vi "Left Camera Loop (SubVI).vi"   [LabVIEW 2015]
uses:
  <vilib>/myRIO/Instrument Drivers/Onboard IO/SPI/typedefs/SPI User Configuration.ctl
  <vilib>/myRIO/Common/Instrument Driver Framework/myRIO v1.0/SPI/typedefs/SPI Clock Phase.ctl
  <vilib>/myRIO/Common/Instrument Driver Framework/myRIO v1.0/SPI/typedefs/SPI Clock Polarity.ctl
  <vilib>/myRIO/Common/Instrument Driver Framework/myRIO v1.0/SPI/typedefs/SPI Data Direction.ctl
  <vilib>/myRIO/Common/Instrument Driver Framework/myRIO v1.0/SPI/typedefs/SPI Frame Length.ctl
  <vilib>/Utility/error.llb/Error Cluster From Error Code.vi
  <vilib>/myRIO/Common/Instrument Driver Framework/myRIO v1.0/SPI/vis/myRIO v1.0 Configure SPI.vi
  Left Variables.vi
  <vilib>/myRIO/Instrument Drivers/Onboard IO/SPI/SPI.lvlib
types:
  T1 = typedef "SPI.lvlib/SPI User Configuration.ctl" = cluster{"Frequency [Hz]":dbl, "Clock Phase":T2, "Clock Polarity":T3, "Data Direction":T4, "Frame Length":T5}
  T2 = typedef "SPI Clock Phase.ctl" = enum8{"Leading", "Trailing"}
  T3 = typedef "SPI Clock Polarity.ctl" = enum8{"Low", "High"}
  T4 = typedef "SPI Data Direction.ctl" = enum8{"Most significant bit first", "Least significant bit first"}
  T5 = typedef "SPI Frame Length.ctl" = u8
  T6 = typedef "SPI.lvlib/SPI Reference.ctl" = cluster{"myRIO Reference":T7, "SPI Channels Enum":T11, "SPI Configuration":T12}
  T7 = typedef "myRIO Generic Hardware Reference.ctl" = cluster{"myRIO Model":T8, "myRIO Hardware Reference":T9}
  T8 = typedef "Hardware Version Enum.ctl" = enum16{"Unknown", "myRIO-1900", "myRIO-1950", "roboRIO"}
  T9 = typedef "myRIO v1.0 Reference.ctl" = cluster{"Generic FPGA Reference":T10, "Allow multiple opens":bool}
  T10 = typedef "Generic FPGA Reference.ctl" = refnum<k20>
  T11 = typedef "SPI Channels Enum.ctl" = enum16{"Not Connected", "A/SPI", "B/SPI", "SPI/SPI"}
  T12 = typedef "SPI.lvlib/SPI Configuration.ctl" = cluster{"Frequency [Hz]":dbl, "Clock Phase":T2, "Clock Polarity":T3, "Data Direction":T4, "Frame Length":T5}
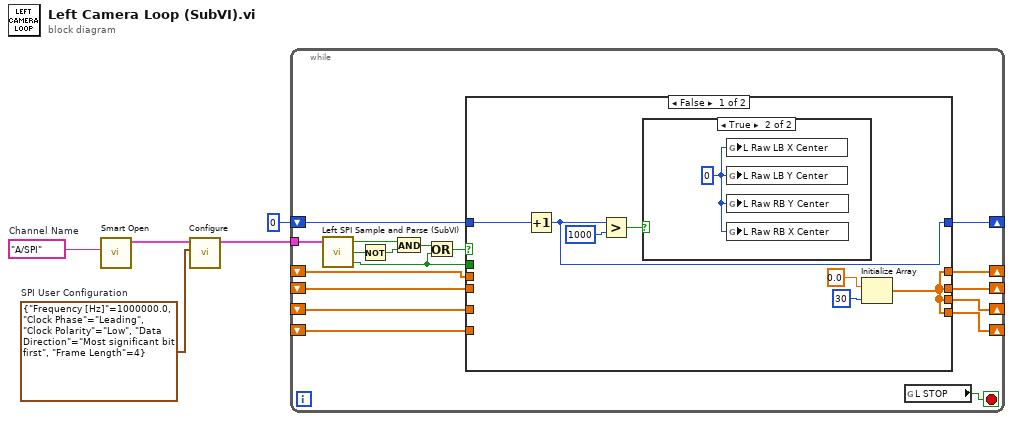
[diagram p0: block diagram]
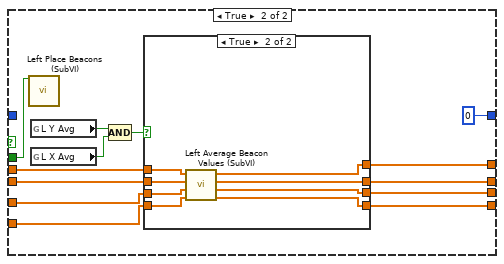
[diagram p3: hidden frame]
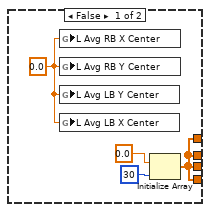
[diagram p4: hidden frame]
diagram:
  w3 = T1 {"Frequency [Hz]"=1000000.0, "Clock Phase"=enum."Leading", "Clock Polarity"=enum."Low", "Data Direction"=enum."Most significant bit first", "Frame Length"=4}  # SPI User Configuration
  w4 = tag "A/SPI"  # Channel Name
  n1 = call <vilib>:"Smart Open.vi"("Channel Name"=w4) -> ("SPI Ref Out"=w2:T6)  [unwired: 9 in, 1 out]
  n2 = call <vilib>:"Configure.vi"("SPI User Configuration"=w3, "SPI Ref In"=w2) -> ("SPI Ref Out"=w1:T6)  [unwired: 8 in, 1 out]
  n3 = while {
    shift-right: [w18] -> _
    shift-left: _ -> [w22]
    shift-right: [w17] -> _
    shift-left: _ -> [w21]
    shift-right: [w16] -> _
    shift-left: _ -> [w20]
    shift-right: [w19] -> _
    shift-left: _ -> [w23]
    shift-right: [w11] -> _
    shift-left: 0 -> [w12]
    tunnel: w1 -> [w9]
    stop <- w10 stop-if-true
    n4 = call "Left SPI Sample and Parse (SubVI).vi"("SPI Ref In"=w9) -> ("Two Beacons Seen?"=w8:bool, "o2 Checksum OK?"=w6:bool, "o1 Checksum OK?"=w7:bool)  [unwired: 2 in]
    n5 = Not(x=w6) -> (.not. x?=w15:bool)
    n6 = And(x=w7, y=w15) -> (x .and. y?=w13:bool)
    n7 = Or(x=w13, y=w8) -> (x .or. y?=w14:bool)
    n8 = case shown="False" w14 {
      tunnel: w23 -> [_ w44]
      tunnel: w22 -> [_ w43]
      tunnel: w21 -> [_ w42]
      tunnel: w20 -> [_ w41]
      tunnel: [w28 w40] -> w19
      tunnel: [w28 w39] -> w18
      tunnel: [w28 w38] -> w17
      tunnel: [w28 w37] -> w16
      tunnel: w8 -> [_ w33]
      tunnel: w12 -> [w26 _]
      tunnel: [w25 0] -> w11
      frame False {
        n9 = Increment(x=w26) -> (x+1=w25:i32)
        n10 = Greater?(x=w25, y=1000) -> (0:w27:bool)
        n11 = case shown="True" w27 {
          frame False {
          }
          frame True {
            w31 = u16 0
            n12 = global write "Left Variables.vi" "L Raw LB X Center"(w31) -> ()
            n13 = global write "Left Variables.vi" "L Raw LB Y Center"(w31) -> ()
            n14 = global write "Left Variables.vi" "L Raw RB Y Center"(w31) -> ()
            n15 = global write "Left Variables.vi" "L Raw RB X Center"(w31) -> ()
          }
        }
        n16 = Initialize Array(0.0 ("element"), 30 ("dimension size")) -> (w28:dbl[])
      }
      frame True {
        n17 = call "Left Place Beacons (SubVI).vi"("Two Beacons Seen"=w33) -> ()  [unwired: 15 in]
        n18 = global read "Left Variables.vi" "L Y Avg"() -> (w36:bool)
        n19 = global read "Left Variables.vi" "L X Avg"() -> (w35:bool)
        n20 = Compound Arithmetic op=AND(w36, w35) -> (w34:bool)
        n21 = case shown="True" w34 {
          tunnel: w44 -> [_ w56]
          tunnel: w43 -> [_ w54]
          tunnel: w42 -> [_ w52]
          tunnel: w41 -> [_ w50]
          tunnel: [w46 w55] -> w40
          tunnel: [w46 w53] -> w39
          tunnel: [w46 w51] -> w38
          tunnel: [w46 w49] -> w37
          frame False {
            w45 = 0.0
            n22 = global write "Left Variables.vi" "L Avg RB X Center"(w45) -> ()
            n23 = global write "Left Variables.vi" "L Avg RB Y Center"(w45) -> ()
            n24 = global write "Left Variables.vi" "L Avg LB Y Center"(w45) -> ()
            n25 = global write "Left Variables.vi" "L Avg LB X Center"(w45) -> ()
            n26 = Initialize Array(0.0 ("element"), 30 ("dimension size")) -> (w46:dbl[])
          }
          frame True {
            n27 = call "Left Average Beacon Values (SubVI).vi"("RB Y Center Array"=w50, "RB X Center Array"=w52, "LB Y Center Array"=w54, "LB X Center Array"=w56) -> ("RB Y Center Array"=w49:dbl[], "RB X Center Array"=w51:dbl[], "LB Y Center Array"=w53:dbl[], "LB X Center Array"=w55:dbl[])  [unwired: 4 in]
          }
        }
      }
    }
    n28 = global read "Left Variables.vi" "L STOP"() -> (w10:bool)
  }
